vi "StandAloneTransient_FileFolderCreation_V2.vi"(8 "error in (no error)":errorcluster, 11 "base path":path) -> (0 "error out":errorcluster, 1 "Latchup_or_Transient":bool, 2 "BinaryRefObjects":T1, 3 "ForcedResetTimingPath":path, 4 "IndicatorOutputs":cluster{"name or relative path":string, string}, 5 "OscopeParamPath":path)   [LabVIEW 2019]
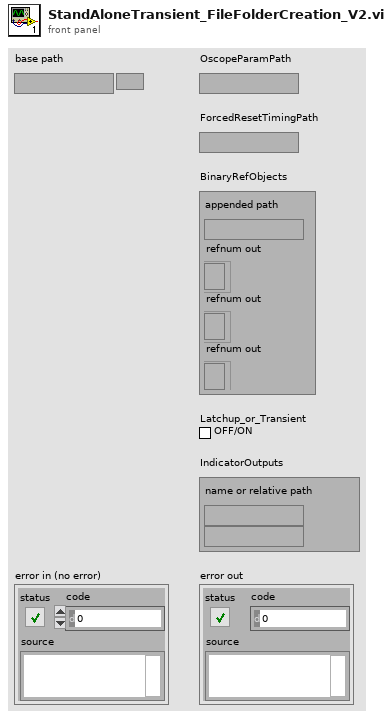
[diagram p1: front panel]
types:
  T1 = cluster{"appended path":path, "refnum out":refnum<file>, "refnum out":refnum<file>, "refnum out":refnum<file>}
  T2 = enum16{"open", "replace", "create", "open or create", "replace or create", "replace or create with confirmation"}
  T3 = enum16{"Left Button", "Center Button", "Right Button", "Window Close"}
  T4 = cluster{"created path":path, "refnum out":refnum<file>, "refnum out":refnum<file>, "refnum out":refnum<file>}
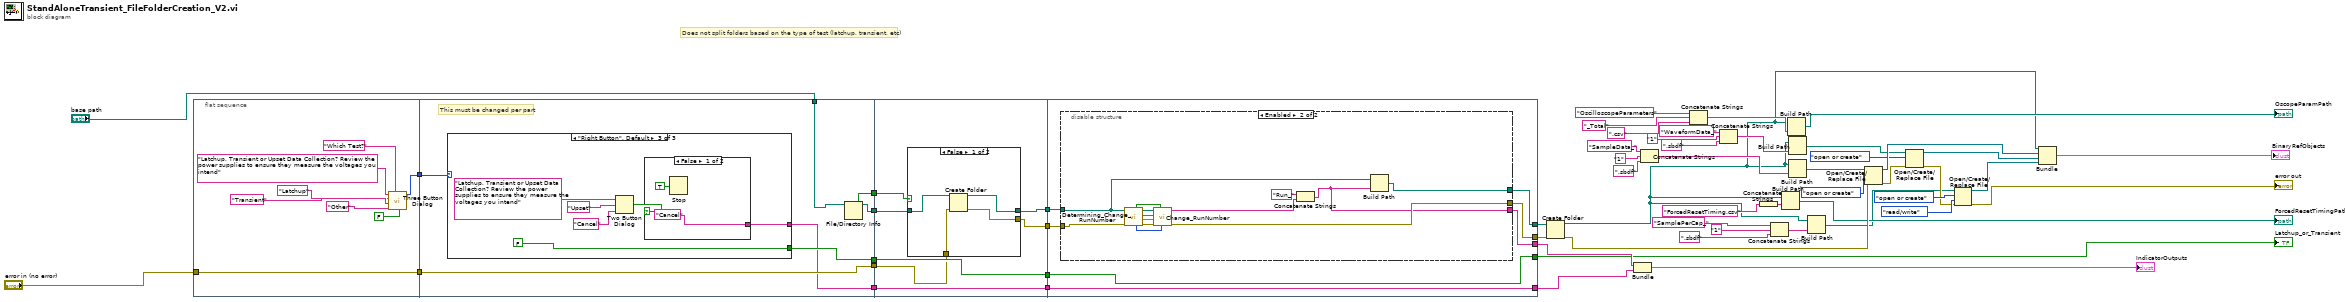
[diagram p0: block diagram]
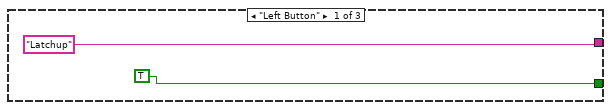
[diagram p2: hidden frame]
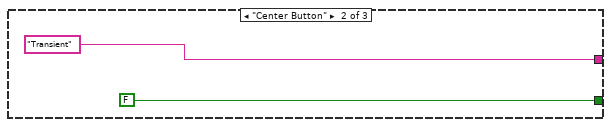
[diagram p3: hidden frame]
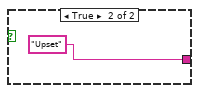
[diagram p4: hidden frame]
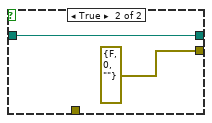
[diagram p5: hidden frame]
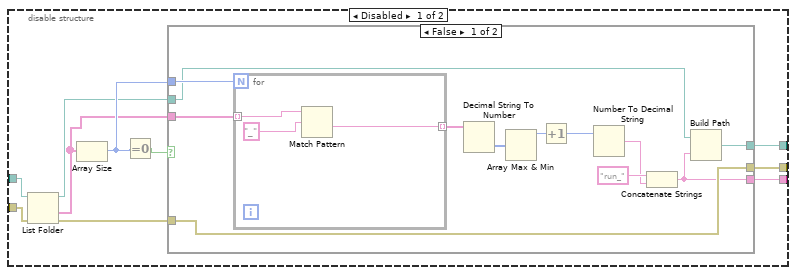
[diagram p6: hidden frame]
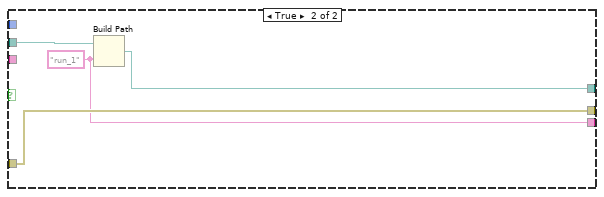
[diagram p7: hidden frame]
diagram:
  # "Does not split folders based on the type of test (latchup, transient, etc)"
  n1 = flat-sequence {
    tunnel: [w57] -> w55
    tunnel: [w56] -> w54
    tunnel: "error in (no error)" -> [w56]
    tunnel: w55 -> [w70]
    tunnel: [w69] -> w53
    tunnel: [w68] -> w52
    tunnel: [w67] -> w51
    tunnel: [w66] -> w50
    tunnel: w54 -> [w66]
    tunnel: "base path" -> [w64]
    tunnel: [w65] -> w49
    tunnel: w53 -> [w90]
    tunnel: w52 -> [w89]
    tunnel: [w88] -> w48
    tunnel: [w87] -> w47
    tunnel: w51 -> [w86]
    tunnel: [w86] -> w46
    tunnel: w50 -> [w85]
    tunnel: [w84] -> w45
    tunnel: w49 -> [w84]
    tunnel: w48 -> [w103]
    tunnel: w47 -> [w99]
    tunnel: [w102] -> w31
    tunnel: [w101] -> w32
    tunnel: [w100] -> w42
    tunnel: [w98] -> w6
    tunnel: w46 -> [w98]
    tunnel: [w97] -> w43
    tunnel: w45 -> [w97]
    frame #0 {
      n2 = call <vilib>:"Three Button Dialog.vi"("Allow user to close window? (TRUE)"=FALSE, "Window Title (\"\")"="Which Test?" ("Window Title (\"\")"), "Right Button Text (\"Cancel\")"="Other" ("Right Button Text (\"Cancel\")"), "Center Button Text (\"No\")"="Transient" ("Center Button Text (\"No\")"), "Left Button Text (\"Yes\")"="Latchup" ("Left Button Text (\"Yes\")"), "message"="Latchup, Transient or Upset Data Collection? Review the power supplies to ensure they measure the voltages you intend") -> ("Which Button?"=w57:T3)  [unwired: 5 in]
    }
    frame #1 {
      # "This must be changed per part"
      n3 = case shown="\"Right Button\", Default" w70 {
        tunnel: ["Latchup" "Transient" w75] -> w65
        tunnel: [TRUE FALSE FALSE] -> w67
        frame "Left Button" {
        }
        frame "Center Button" {
        }
        frame "Right Button", Default {
          n4 = Two Button Dialog(message="Latchup, Transient or Upset Data Collection? Review the power supplies to ensure they measure the voltages you intend", 1:"Cancel" ("F button name (\"Cancel\")"), 2:"Upset" ("T button name (\"OK\")")) -> (T button?=w76:bool)
          n5 = case shown="False" w76 {
            tunnel: ["Cancel" ("F button name (\"Cancel\")") "Upset" ("T button name (\"OK\")")] -> w75
            frame False {
              n6 = Stop(stop? (T)=TRUE) -> ()
            }
            frame True {
            }
          }
        }
      }
      n7 = File/Directory Info(path=w64) -> (path out=w68:path, directory=w69:bool)  [unwired: 1 in, 5 out]
    }
    frame #2 {
      n8 = case shown="False" w90 {
        tunnel: w89 -> [w94 w96]
        tunnel: [w93 w96] -> w87
        tunnel: [w92 errorcluster {"status"=FALSE, "code"=0, "source"=""} ("error out")] -> w88
        tunnel: w85 -> [w91 _]
        frame False {
          n9 = Create Folder(path (use dialog)=w94, error in=w91) -> (created path=w93:path, error out=w92:errorcluster)  [unwired: 1 in, 1 out]
        }
        frame True {
        }
      }
    }
    frame #3 {
      n10 = disable-structure shown="Enabled" {
        disable-tunnel: w103 -> [w109 w140]
        disable-tunnel: [w108 w134] -> w102
        disable-tunnel: [w107 w136] -> w101
        disable-tunnel: [w106 w133] -> w100
        disable-tunnel: w99 -> [w104 w135]
        frame Disabled {
          n11 = List Folder(path=w104, error in=w109) -> (path out=w105:path, folder names=w110:string[], error out=w111:errorcluster)  [unwired: 2 in, 1 out]
          n12 = Array Size(array=w110) -> (size(s)=w113:i32)
          n13 = Equal To 0?(x=w113) -> (x = 0?=w112:bool)
          n14 = case shown="False" w112 {
            tunnel: w105 -> [w117 w132]
            tunnel: w110 -> [w124 _]
            tunnel: w111 -> [w115 w130]
            tunnel: w113 -> [w125 _]
            tunnel: [w116 w131] -> w108
            tunnel: [w115 w130] -> w107
            tunnel: [w114 w129] -> w106
            frame False {
              n15 = for {
                N: w125 -> [_]
                tunnel: w124 -> [w128] mode=indexing
                tunnel: [w126] -> w123 mode=indexing
                n16 = Match Pattern(string=w128, regular expression="_" ("search string/char (-)")) -> (after substring=w126:string)  [unwired: 1 in, 3 out]
              }
              n17 = Decimal String To Number(string=w123) -> (number=w122:i32[])  [unwired: 2 in, 1 out]
              n18 = Array Max & Min(array=w122) -> (max value=w121:i32)  [unwired: 3 out]
              n19 = Increment(x=w121) -> (x+1=w119:i32)
              n20 = Number To Decimal String(number=w119) -> (decimal integer string=w118:string)  [unwired: 1 in]
              n21 = Concatenate Strings("run_" ("string"), w118) -> (w114:string)
              n22 = Build Path(base path=w117, name or relative path=w114) -> (appended path=w116:path)
            }
            frame True {
              w129 = "run_1" ("name or relative path")
              n23 = Build Path(base path=w132, name or relative path=w129) -> (appended path=w131:path)
            }
          }
        }
        frame Enabled {
          n24 = call "Determining_Change_RunNumber.vi"("error in"=w140, "Run Folder Parent Directory"=w135) -> ("error out"=w141:errorcluster, "Array"=w142:dbl[], "String"=w143:string, "path out"=w144:path, "Proposed Run Number"=w145:i32, "T button?"=w139:bool)  [unwired: 4 in]
          n25 = call "Change_RunNumber.vi"("Valid Run Number"=w145, "Changing the run number?"=w139, "error in (no error)"=w141, "Array"=w142, "String in"=w143, "path in"=w144) -> ("error out"=w136:errorcluster, "String out"=w137:string)  [unwired: 4 in]
          n26 = Concatenate Strings("Run_" ("string"), w137) -> (w133:string)
          n27 = Build Path(base path=w135, name or relative path=w133) -> (appended path=w134:path)
        }
      }
    }
  }
  n28 = Create Folder(path (use dialog)=w31, error in=w32) -> (created path=w1:path, error out=w13:errorcluster)  [unwired: 1 in, 1 out]
  n29 = Bundle(w42, "T button name (\"OK\")"=w43) -> (→"IndicatorOutputs":cluster{string, "T button name (\"OK\")":string})  [unwired: 1 in]
  n30 = Concatenate Strings("SampleData_", "1" ("string"), ".sbdf" ("string")) -> (w15:string)
  n31 = Concatenate Strings("OscilloscopeParameters" ("name or relative path"), "_Total" ("string"), ".csv" ("string")) -> (w25:string)
  n32 = Concatenate Strings("WaveformData_" ("name or relative path"), "1" ("string"), ".sbdf" ("string")) -> (w22:string)
  n33 = Concatenate Strings("ForcedResetTiming.csv" ("string")) -> (w33:string)
  n34 = Concatenate Strings("SamplePerCap_", "1" ("string"), ".sbdf" ("string")) -> (w30:string)
  n35 = Build Path(base path=w1, name or relative path=w33) -> (appended path=→"ForcedResetTimingPath":path)
  n36 = Build Path(base path=w1, name or relative path=w25) -> (appended path=→"OscopeParamPath":path)
  n37 = Build Path(base path=w1, name or relative path=w22) -> (appended path=w11:path)
  n38 = Build Path(base path=w1, name or relative path=w15) -> (appended path=w14:path)
  n39 = Build Path(base path=w1, name or relative path=w30) -> (appended path=w2:path)
  n40 = Open/Create/Replace File ("Open/Create/Replace File - first sample binary")(file path (use dialog)=w14, error in=w13, operation (0:open)=T2."open or create") -> (refnum out=w36:refnum<file>, error out=w9:errorcluster)  [unwired: 3 in, 1 out]
  n41 = Open/Create/Replace File ("Open/Create/Replace File - first timestamp binary")(file path (use dialog)=w11, error in=w9, operation (0:open)=T2."open or create") -> (refnum out=w37:refnum<file>, error out=w3:errorcluster)  [unwired: 3 in, 1 out]
  n42 = Open/Create/Replace File ("Open/Create/Replace File - oscope parameters")(file path (use dialog)=w2, error in=w3, operation (0:open)=T2."open or create", access (0:read/write)=enum16{"read/write", "read-only", "write-only"}."read/write") -> (refnum out=w38:refnum<file>, error out=→"error out":errorcluster)  [unwired: 2 in, 1 out]
  n43 = Bundle("created path"=w1, "refnum out"=w36, "refnum out"=w37, "refnum out"=w38) -> (→"BinaryRefObjects":T4)  [unwired: 1 in]
  "Latchup_or_Transient" <- w6
